vi "CORE2_SERIAL_STUDY.vi"() -> ()   [LabVIEW 2017]
uses:
  <vilib>/Instr/_visa.llb/VISA Configure Serial Port (Instr).vi
panel:
  in  "정지 버튼 2":bool
  in  "정지 버튼":bool
  out "루프타임":u32
  out "버퍼 읽기":string
  out "Serial Settings:Number of Bytes at Serial Port":u32
  in  "baud rate (9600) 2":u32=9600 caption="보 전송속도(9600)"
  in  "VISA resource name 2":refnum<visa-resource-name> caption="VISA 리소스 이름"
  in  "baud rate (9600)":u32=9600 caption="보 전송속도(9600)"
  in  "VISA resource name":refnum<visa-resource-name> caption="VISA 리소스 이름"
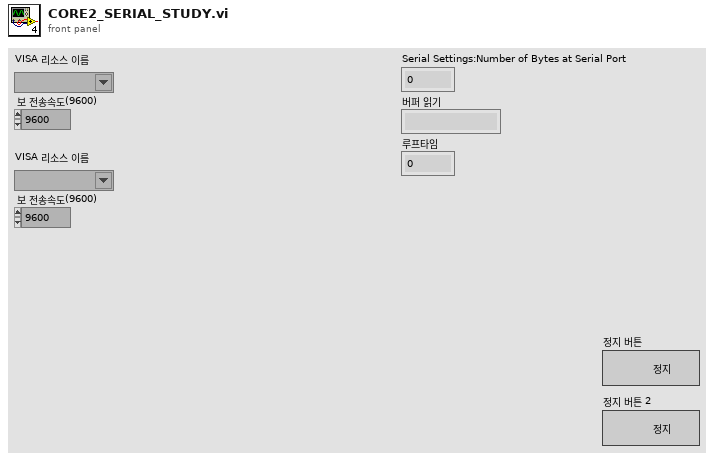
[diagram p1: front panel]
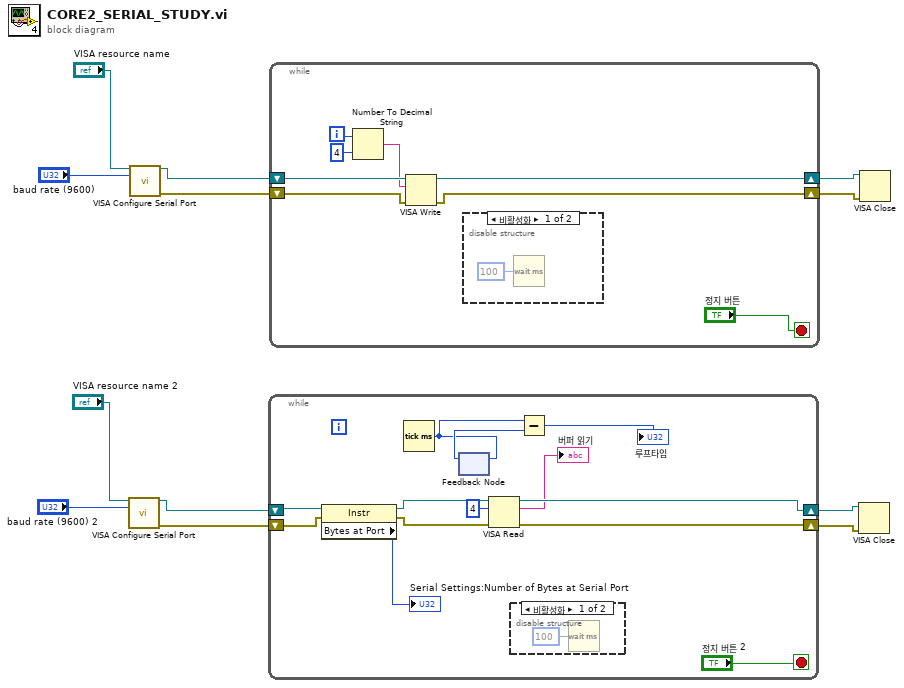
[diagram p0: block diagram]
diagram:
  n1 = call-poly "VISA Configure Serial Port"("VISA resource name"="VISA resource name 2", "baud rate (9600)"="baud rate (9600) 2") -> ("VISA resource name out"=w4:refnum<visa-resource-name>, "error out"=w3:errorcluster)  [unwired: 7 in, 5 out]
  n2 = call-poly "VISA Configure Serial Port"("VISA resource name"="VISA resource name", "baud rate (9600)"="baud rate (9600)") -> ("VISA resource name out"=w10:refnum<visa-resource-name>, "error out"=w9:errorcluster)  [unwired: 7 in, 5 out]
  n3 = while {
    shift-right: [w19] -> w2
    shift-left: w4 -> [w25]
    shift-right: [w20] -> w1
    shift-left: w3 -> [w24]
    stop <- "정지 버튼 2" stop-if-true
    n4 = property class="Instr"(reference=w25, error in=w24) -> (reference out=w22:refnum<visa-resource-name>, error out=w21:errorcluster, "Bytes at Port"=→"Serial Settings:Number of Bytes at Serial Port":u32)
    n5 = Tick Count (ms)() -> (millisecond timer value=w16:u32)
    n6 = feedback-in #1(w16) -> ()
    n7 = feedback #1() -> (w17:u32)  [unwired: 1 in]
    n8 = VISA Read(VISA resource name=w22, byte count=u32 4 ("바이트 카운트"), error in (no error)=w21) -> (VISA resource name out=w19:refnum<visa-resource-name>, read buffer=→"버퍼 읽기":string, error out=w20:errorcluster)  [unwired: 1 out]
    n9 = disable-structure shown="비활성화" {
      frame Disabled {
        n10 = Wait (ms)(milliseconds to wait=u32 100 ("대기 시간 (ms)")) -> ()  [unwired: 1 out]
      }
      frame Enabled {
      }
    }
    n11 = Subtract(x=w16, y=w17) -> (x-y=→"루프타임":u32)
  }
  n12 = while {
    shift-right: [w29] -> w8
    shift-left: w10 -> [w34]
    shift-right: [w28] -> w7
    shift-left: w9 -> [w30]
    i -> [w33]
    stop <- "정지 버튼" stop-if-true
    n13 = Number To Decimal String(number=w33, width (-)=i16 4 ("폭(-)")) -> (decimal integer string=w31:string)
    n14 = VISA Write(VISA resource name=w34, write buffer=w31, error in (no error)=w30) -> (VISA resource name out=w29:refnum<visa-resource-name>, error out=w28:errorcluster)  [unwired: 1 out]
    n15 = disable-structure shown="비활성화" {
      frame Disabled {
        n16 = Wait (ms)(milliseconds to wait=u32 100 ("대기 시간 (ms)")) -> ()  [unwired: 1 out]
      }
      frame Enabled {
      }
    }
  }
  n17 = VISA Close(VISA resource name=w2, error in (no error)=w1) -> ()  [unwired: 1 out]
  n18 = VISA Close(VISA resource name=w8, error in (no error)=w7) -> ()  [unwired: 1 out]
